vi "UtilityLib.CSV read.vi"(1 "file (use dialog)":path, 5 "error in":errorcluster) -> (15 "CSVArray":string[][](array[string]), 19 "error out":errorcluster)   [LabVIEW 2015, in "UtilityLib.lvlib"]
doc: "Reads information about from a CSV file and converts that information into a 2-dim array. The fields in the CSV file may be embedded in double quotes (\") . However, the information embedded in double quotes may not contain special characters like double quotes, carriage returns or line feeds."
uses:
  UtilityLib.lvlib
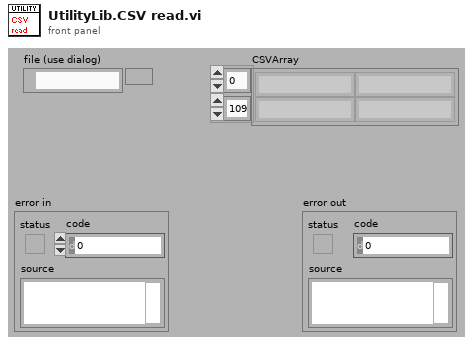
[diagram p1: front panel]
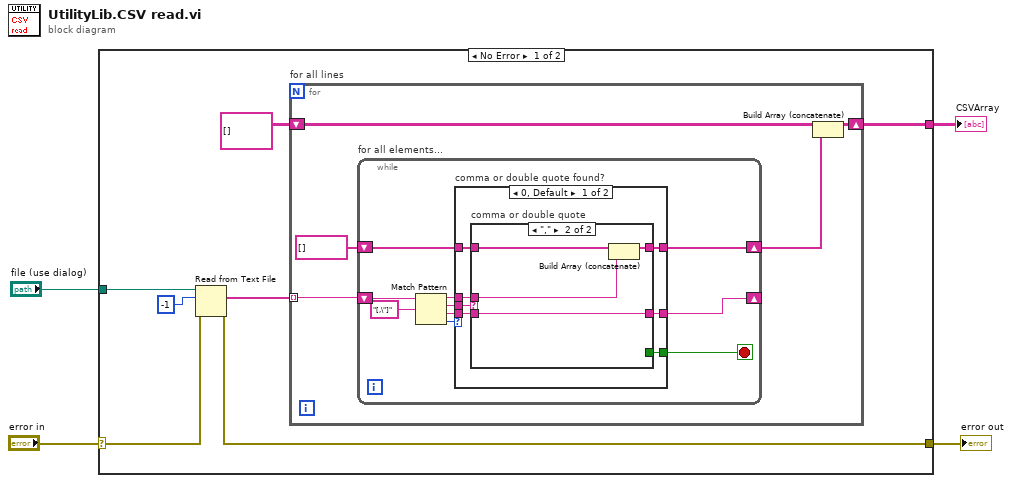
[diagram p0: block diagram]
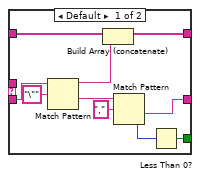
[diagram p2: hidden frame]
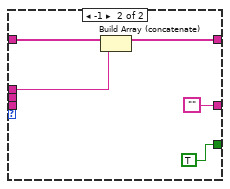
[diagram p3: hidden frame]
diagram:
  n1 = case shown="No Error" "error in" {
    selector: "error in" -> [w9 w53]
    tunnel: [w11 w53] -> w4
    tunnel: "file (use dialog)" -> [w10 _]
    tunnel: [w5 _] -> w1
    frame No Error {
      n2 = Read from Text File(file (use dialog)=w10, count=-1, error in=w9) -> (text=w7:string[], error out=w11:errorcluster)  [unwired: 1 in, 2 out]
      n3 = for "for all lines" {
        tunnel: w7 -> [w13] mode=indexing
        shift-right: [w14] -> w5
        shift-left: string[][] [] -> [w15]
        n4 = while "for all elements..." {
          shift-right: [w21] -> _
          shift-left: w13 -> [w26]
          shift-right: [w19] -> w12
          shift-left: string[] [] -> [w20]
          stop <- w17 stop-if-true
          n5 = Match Pattern(string=w26, regular expression="[,\"]") -> (before substring=w23:string, match substring=w24:string, after substring=w22:string, offset past match=w18:i32)  [unwired: 1 in]
          n6 = case "comma or double quote found?" shown="0, Default" w18 {
            tunnel: w24 -> [w33 _]
            tunnel: w23 -> [w32 w52]
            tunnel: w22 -> [w31 _]
            tunnel: [w30 "" ("Empty String Constant")] -> w21
            tunnel: w20 -> [w29 w49]
            tunnel: [w28 w48] -> w19
            tunnel: [w27 TRUE] -> w17
            frame 0, Default {
              n7 = case "comma or double quote" shown="\",\"" w33 {
                tunnel: w32 -> [_ w44]
                tunnel: w31 -> [w42 w47]
                tunnel: [w40 w47] -> w30
                tunnel: w29 -> [w38 w46]
                tunnel: [w37 w45] -> w28
                tunnel: [w35 _] -> w27
                frame Default {
                  n8 = Match Pattern(string=w42, regular expression="\"") -> (before substring=w39:string, after substring=w41:string)  [unwired: 1 in, 2 out]
                  n9 = Build Array (concatenate)(w38, w39) -> (w37:string[])
                  n10 = Match Pattern(string=w41, regular expression=",") -> (after substring=w40:string, offset past match=w34:i32)  [unwired: 1 in, 2 out]
                  n11 = Less Than 0?(x=w34) -> (x < 0?=w35:bool)
                }
                frame "," {
                  n12 = Build Array (concatenate)(w46, w44) -> (w45:string[])
                }
              }
            }
            frame -1 {
              n13 = Build Array (concatenate)(w49, w52) -> (w48:string[])
            }
          }
        }
        n14 = Build Array (concatenate)(w15, w12) -> (w14:string[][])
      }
    }
    frame Error {
    }
  }
  "error out" <- w4
  "CSVArray" <- w1
